vi "Drop Message Core.vi"(11 "Launch Measurement and Wait for Result in":refnum<class "Launch Measurement and Wait for Result.lvclass">) -> ()   [LabVIEW 2015, in "Controller API.lvlib" / "Launch Measurement and Wait for Result.lvclass"]
doc: "(<B>Filename</B>: Actor Framework.lvlib:Message.lvclass:Drop Message Core.vi)\n\nDefines what a message does if it is in the message queue when the queue is released. At this point, the actor has shut down, so it will never process the message.\n\nBy default, this method does nothing. A child class may override it to define behavior. National Instruments provides the Reply Msg class to override this method. This class releases its internal queue, which causes any caller of the Send Message and Wait For Response method to stop waiting and return an error."
uses:
  Launch Measurement and Wait for Result.lvclass
  Launch Measurement and Wait for Result.lvclass/Launch Measurement and Wait for Result.ctl
  <userlib>/Common Components/Controller/Messages/Launch Measurements Message/Launch Measurements Message.lvclass
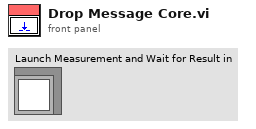
[diagram p1: front panel]
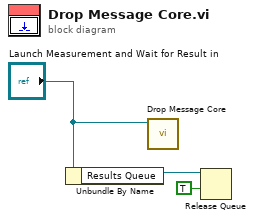
[diagram p0: block diagram]
diagram:
  n1 = Unbundle By Name("Launch Measurement and Wait for Result in") -> ("Results Queue"=w2:refnum<queue>)
  n2 = call-parent "Drop Message Core.vi"("Message in"="Launch Measurement and Wait for Result in") -> ()  [unwired: 11 in]
  n3 = Release Queue(queue=w2, force destroy? (F)=TRUE) -> ()  [unwired: 1 in, 3 out]
